vi "FTW-TestExecutive-ReportResults.vi"(0 "FTW Actor Connector In":refnum<class "FTW-ActorConnector.lvclass">, 5 "Results":T1 {"Start Time" format="%<%Y-%m-%d %H:%M:%S%03u>T"; "Elapsed Time" format="%<%H:%M:%S%3u>t"}, 11 "error in (no error)":errorcluster) -> (4 "FTW Actor Connector":refnum<class "FTW-ActorConnector.lvclass">, 6 "Response":string, 14 "Roundtrip Time":dbl format="%.6fsec", 15 "error out":errorcluster)   [LabVIEW 2015]
doc: "This VI is intended to be used <b>only by test steps</b> to report their results to the Test Executive"
uses:
  source/actor/Connector/FTW-ActorConnector.lvclass
  FTW-TestExecutive-Results.ctl
  source/container/FTW-Container.lvclass
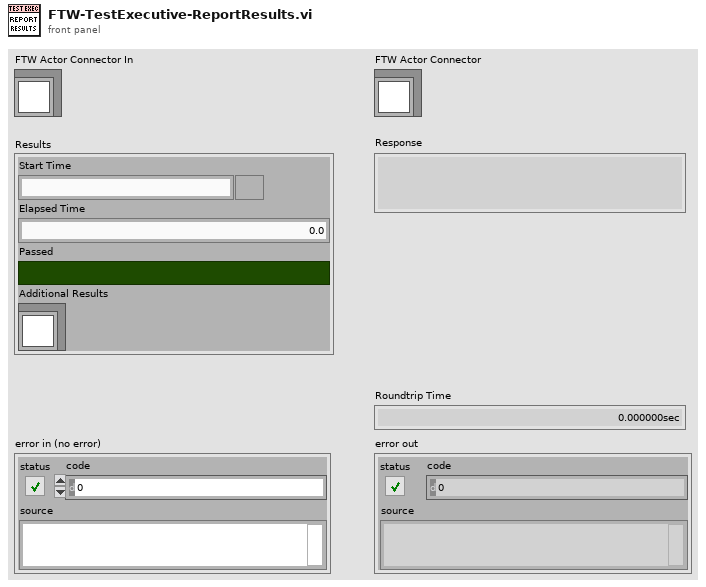
[diagram p1: front panel]
types:
  T1 = typedef "FTW-TestExecutive-Results.ctl" = cluster{"Start Time":timestamp, "Elapsed Time":dbl, "Passed":bool, "Additional Results":refnum<class "FTW-Container.lvclass">}
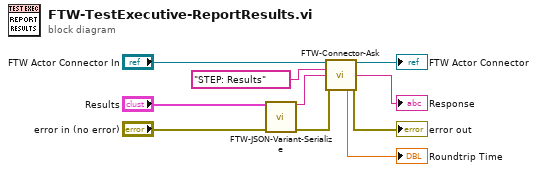
[diagram p0: block diagram]
diagram:
  n1 = call "FTW-JSON-Variant-Serialize.vi"("Variant"="Results", "error in"="error in (no error)") -> ("JSON String"=w2:string, "error out"=w3:errorcluster)  [unwired: 12 in]
  n2 = call "FTW-Connector-Ask.vi"("FTW Actor Connector"="FTW Actor Connector In", "Request Header"="STEP: Results", "Request Body"=w2, "error in"=w3) -> ("FTW Actor Connector out"=→"FTW Actor Connector":refnum<class "FTW-ActorConnector.lvclass">, "Response Body"=→"Response":string, "Roundtrip Time"=→"Roundtrip Time":dbl, "error out"=→"error out":errorcluster)  [unwired: 6 in, 2 out]
